vi "MODBUS  SLAVE.vi"() -> (3 "values to write":u16[](array[numeric]) caption="待写入值")   [LabVIEW 2016]
uses:
  <vilib>/NI/Modbus Library/Data Model/Device Data Model.lvclass
  <vilib>/NI/Modbus Library/API/Wrapper/Create TCP Slave.vi
  <vilib>/NI/Modbus Library/API/Slave/Modbus Slave.lvclass
  <vilib>/ptbypt/NI_PtbyPt.lvlib
  <vilib>/NI/Modbus Library/API/Wrapper/API Main.lvlib
panel:
  out "运行周期":u16[](array[numeric])
  in  "write operation starting address":u16=100 caption="写操作起始地址"
  out "单仪器启动命令":u16[](array[numeric])
  out "系统启动命令":u16[](array[numeric])
  in  "停止":bool
  out "register values":u16[](array[numeric]) caption="寄存器值"
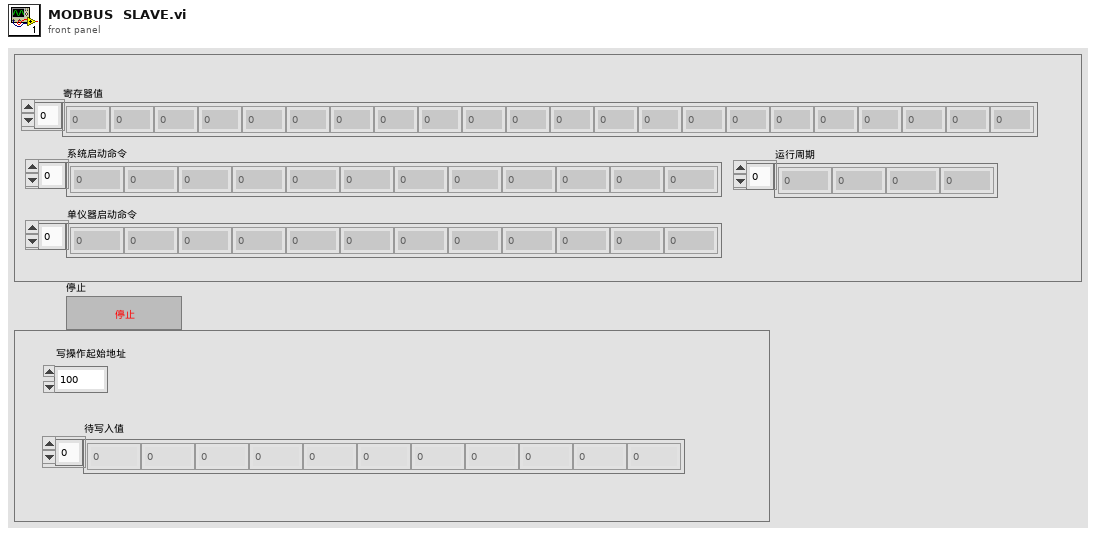
[diagram p1: front panel]
types:
  T1 = cluster{"测量模式":enum16{"水样测量", "标样核查", "零点核查", "跨度核查", "空白测试", "加标回收", "平行样", "校零", "校标"}}
  T2 = cluster{"站号":u16, "量程切换":enum32{"H", "L", "AUTO"}, "控制命令":enum16{"启动测量", "标样核查", "零点核查", "跨度核查", "空白测试", "平行样测试", "加标回收", "空白校准", "标样校准", "初始化（清洗）", "停止测试", "仪器重启", "校时", "模式设置", "测量间隔设置"}, "模式设置":enum16{"待机", "连续模式", "周期模式", "定点模式", "受控模式", "手动模式"}, "测量间隔":u16}
  T3 = cluster{"系统时间":timestamp, "工作状态":enum16{"空闲", "水样测试", "标样核查", "零点核查", "跨度核查", "空白测试", "平行样测试", "加标回收", "空白校准", "标样校准", "初始化（清洗）"}, "测量模式":enum16{"待机", "连续模式", "周期模式", "定点模式", "受控模式", "手动模式"}, "告警代码":enum16{"无告警", "缺试剂告警", "缺水样告警", "缺蒸馏水告警", "缺标液告警", "仪表漏液告警", "标定异常告警", "超量程告警", "加热异常", "低试剂预警", "超上限告警", "超下限告警", "仪表内部其他异常", "滴定异常告警", "电极异常告警", "量程切换告警", "参数设置告警", "PH电极电位异常", "电导率电极异常", "浊度光度异常", "溶解氧电极异常", "溶解氧光强异常", "温度异常告警", "PH异常告警", "溶解氧异常告警", "电导率异常告警", "浊度异常告警", "叶绿素异常告警", "藻密度异常告警", "蓝绿藻异常告警", "ORP异常告警", "氨氮异常告警", "清洁刷异常告警", "SD卡异常告警", "蓝牙异常告警", "Wifi异常告警", "流程异常告警"}, "故障代码":enum16{"无故障", "电机故障", "温度故障", "通讯故障", "滴定故障"}, "日志代码":u16, "软件版本":u16, "F0":sgl, "F1":sgl, "F2":sgl, "F3":sgl, "T":sgl, "H":sgl, "id":u16, "flowid":u16, "量程":u16, "总磷控温温度1":sgl, "营养盐控温温度2":sgl, "ADC":sgl}
  T4 = enum16{"空闲", "水样测试", "标样核查", "零点核查", "跨度核查", "空白测试", "平行样测试", "质控样", "空白校准", "标样校准", "加标回收"}
  T5 = cluster{"当前瓶号：":dbl, "平行样：":dbl, "留样瓶数：":dbl, "每瓶次数：":dbl, "每次留样：":dbl}
  T6 = enum16{"空闲", "水样测试", "标样核查", "零点核查", "跨度核查", "空白测试", "平行样测试", "加标回收", "空白校准", "标样校准", "初始化（清洗）"}
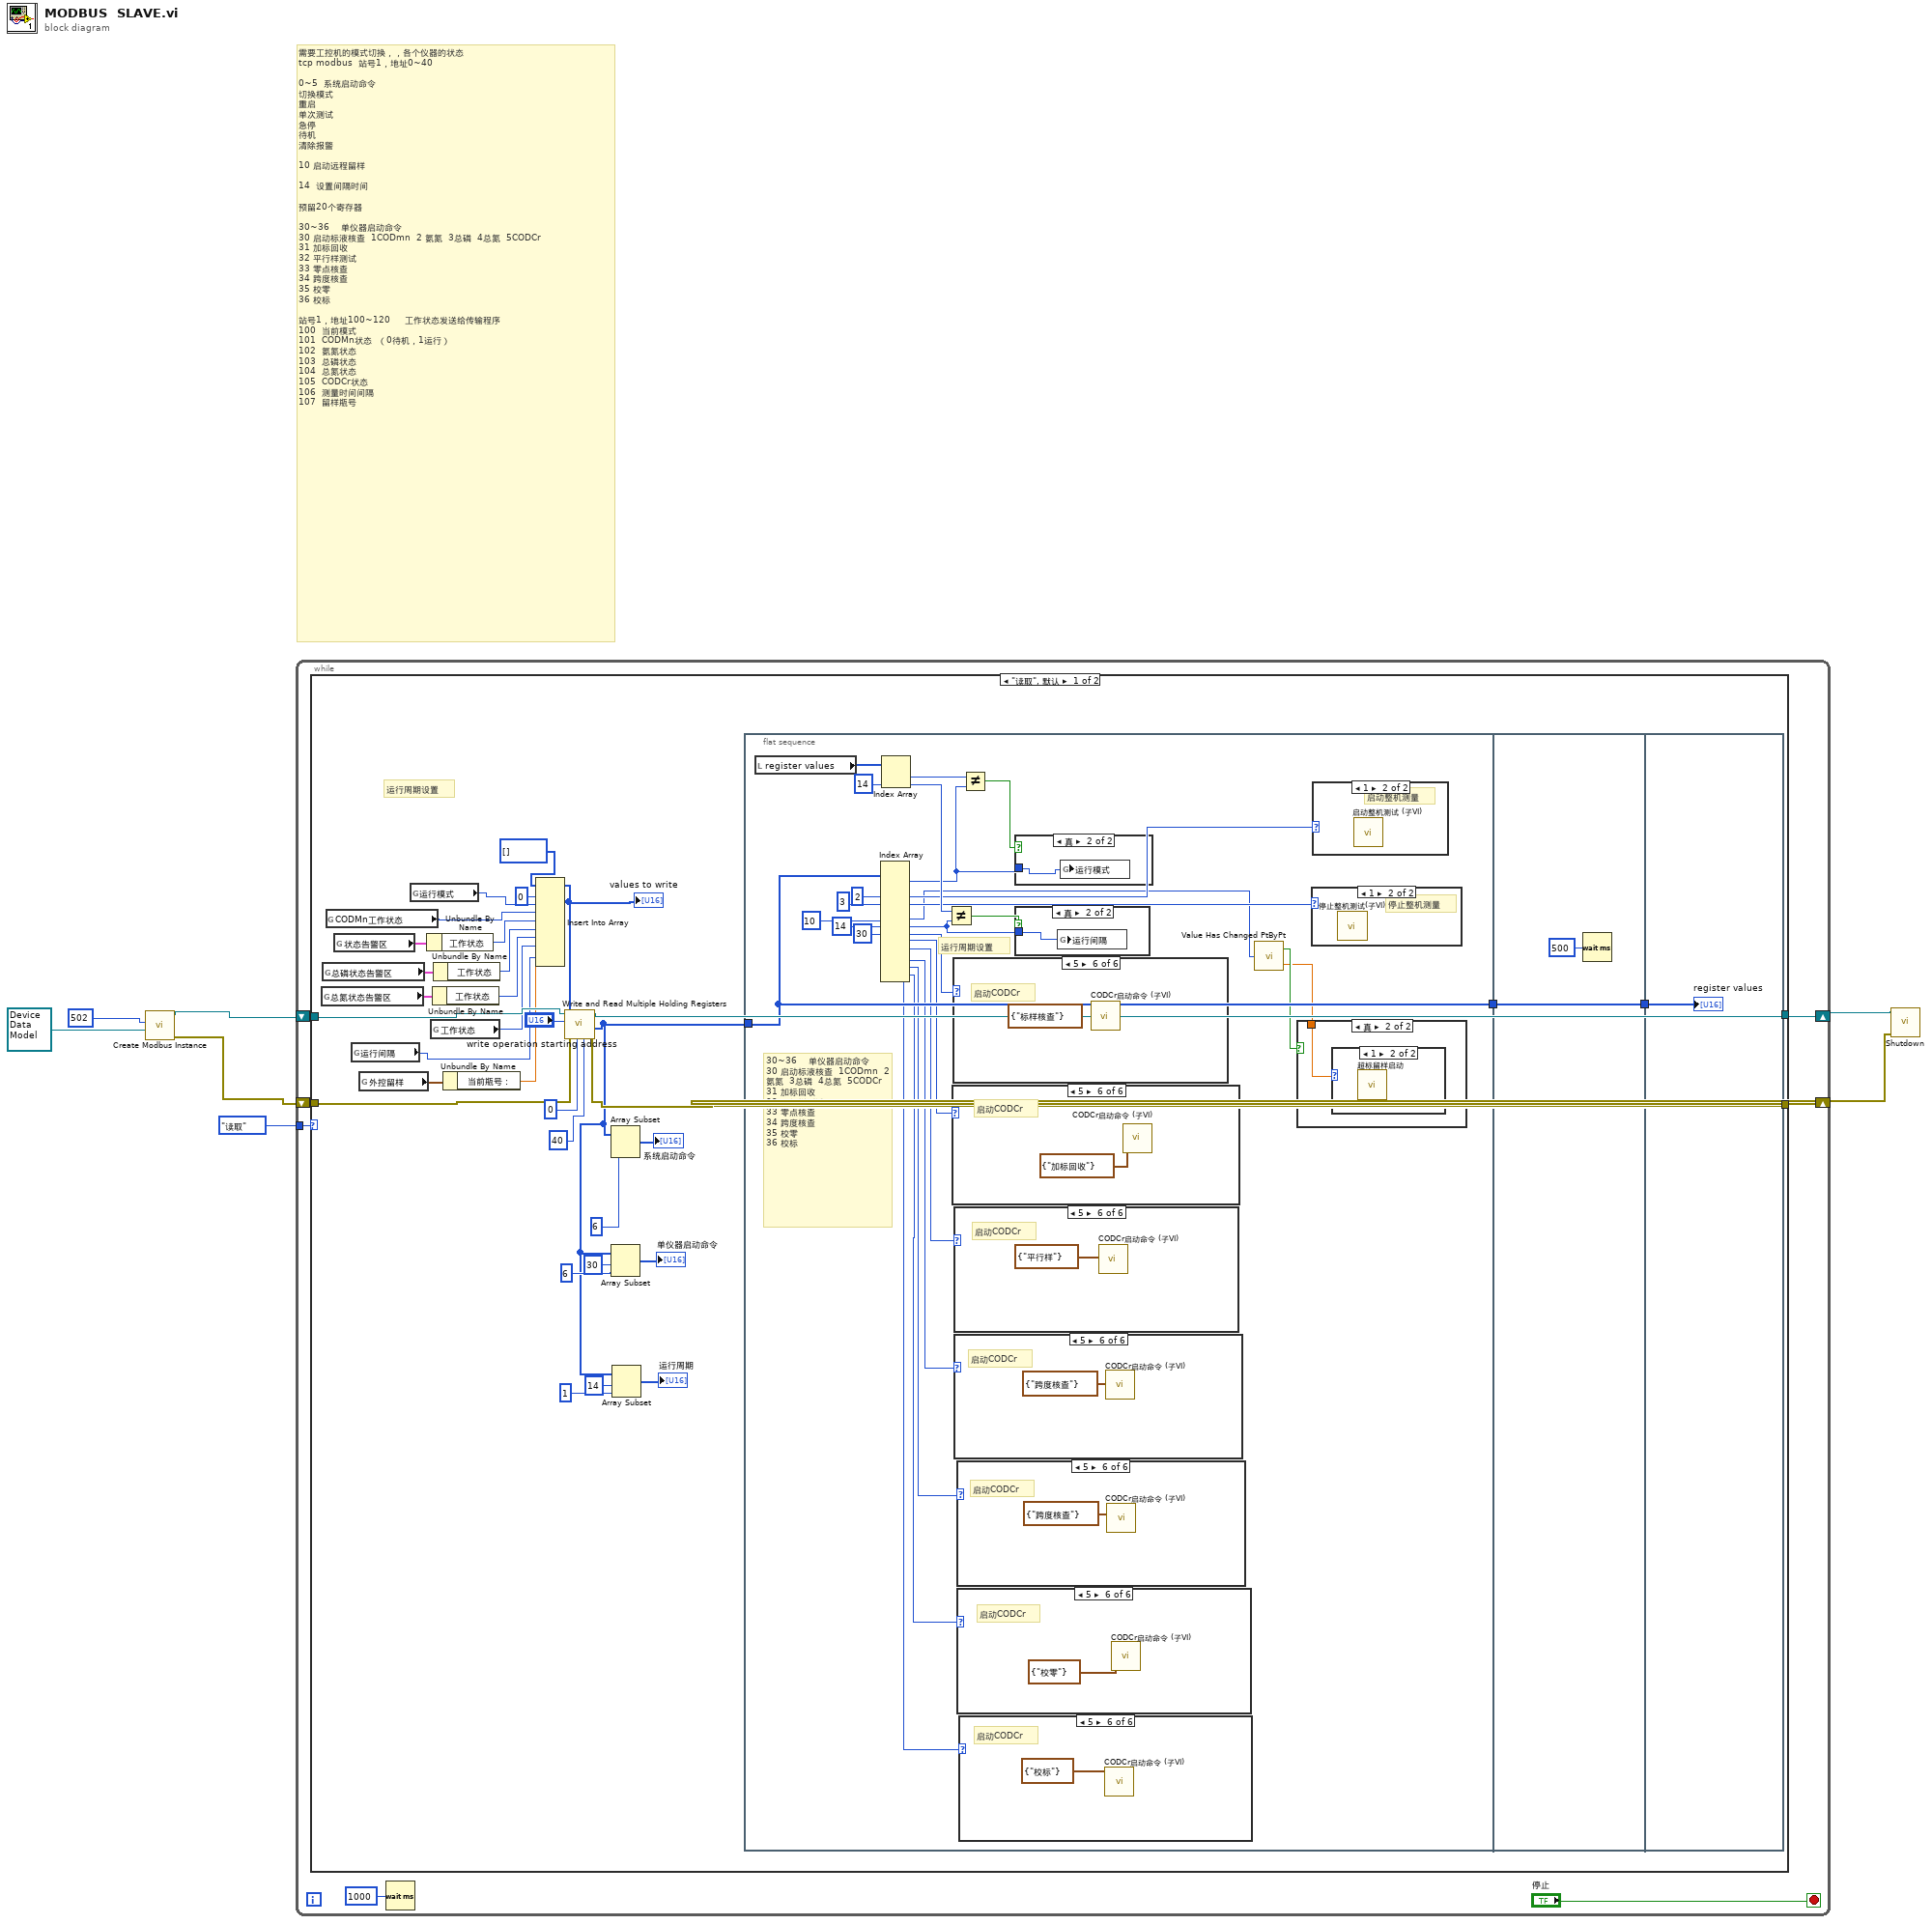
[diagram p0: block diagram]
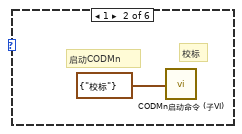
[diagram p5: hidden frame]
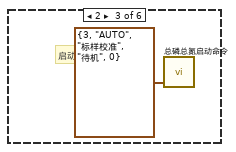
[diagram p6: hidden frame]
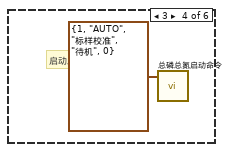
[diagram p7: hidden frame]
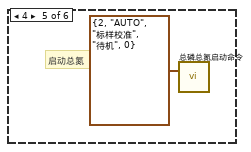
[diagram p8: hidden frame]
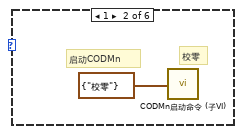
[diagram p10: hidden frame]
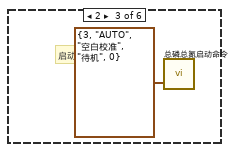
[diagram p11: hidden frame]
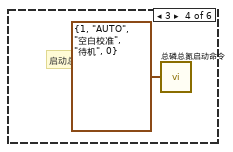
[diagram p12: hidden frame]
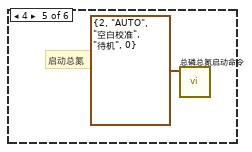
[diagram p13: hidden frame]
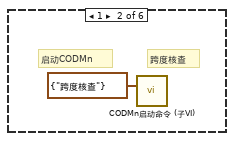
[diagram p15: hidden frame]
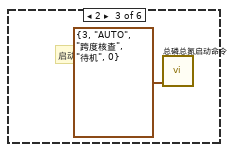
[diagram p16: hidden frame]
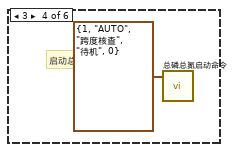
[diagram p17: hidden frame]
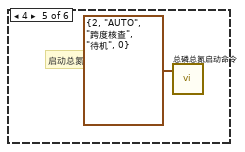
[diagram p18: hidden frame]
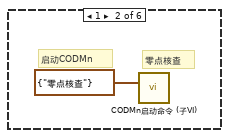
[diagram p20: hidden frame]
diagram:
  # "需要工控机的模式切换，，各个仪器的状态\ntcp modbus  站号1，地址0~40\n\n0~5  系统启动命令\n切换模式\n重启\n单次测试\n急停\n待机\n清除报警\n\n10 启动远程留样\n\n14  设置间隔时间\n\n预留20个寄存器\n\n30~36    单仪器启动命令\n30 启动标液核查  1CODmn  2 氨氮  3总磷  4总氮  5CODCr\n31 加标回收\n32 平行样测试\n33 零点核查\n34 跨度核查\n35 校零\n36 校标\n\n站号1，地址100~120     工作状态发送给传输程序\n100  当前模式\n101  CODMn状态  （0待机，1运行）\n102  氨氮状态\n103  总磷状态\n104  总氮状态\n105  CODCr状态\n106  测量时间间隔\n107  留样瓶号"
  n1 = call-poly <vilib>:"Create Modbus Instance.vi"("device data model"=refnum<class "Device Data Model.lvclass"> refnum, "port (502)"=u16 502) -> ("error out"=w5:errorcluster, "TCP slave instance"=w6:refnum<class "Modbus Slave.lvclass">)  [unwired: 8 in]
  n2 = while {
    shift-right: [w12] -> w2
    shift-left: w6 -> [w14]
    shift-right: [w8] -> w1
    shift-left: w5 -> [w13]
    tunnel: enum16{"读取", "写入"}."读取" -> [w9]
    stop <- "停止" stop-if-true
    n3 = case shown="\"读取\", 默认" w9 {
      tunnel: w14 -> [w43 w116]
      tunnel: w13 -> [w42 w115]
      tunnel: [w38 w116] -> w12
      tunnel: [w39 w115] -> w8
      frame "读取", Default {
        # "运行周期设置"
        n4 = global read "VAR总磷总氮全局变量.vi" "总氮状态告警区"() -> (w22:T3)
        n5 = global read "VAR总磷总氮全局变量.vi" "总磷状态告警区"() -> (w24:T3)
        n6 = global read "COD测量模式全局.vi" "CODMn工作状态"() -> (w20:T4)
        n7 = global read "VAR氨氮全局变量.vi" "状态告警区"() -> (w26:T3)
        n8 = global read "系统设置全局变量.vi" "运行间隔"() -> (w16:i16)
        n9 = global read "超标留样全局.vi" "外控留样"() -> (w18:T5)
        n10 = global read "系统设置全局变量.vi" "运行模式"() -> (w15:enum16{"维护模式", "常规模式", "应急模式", "质控模式"})
        n11 = Unbundle By Name(w26) -> ("工作状态"=w25:T6)
        n12 = global read "CODcr全局变量.vi" "工作状态"() -> (w19:T6)
        n13 = Unbundle By Name(w22) -> ("工作状态"=w21:T6)
        n14 = Unbundle By Name(w24) -> ("工作状态"=w23:T6)
        n15 = Unbundle By Name(w18) -> ("当前瓶号："=w17:dbl)
        n16 = Insert Into Array(array=u16[] [] ("values to write"), index=0 ("索引"), new element #1=w15, new element #2=w20, new element #3=w25, new element #4=w23, new element #5=w21, new element #6=w19, new element #7=w16, new element #8=w17) -> (w34:u16[])
        "values to write" <- w34
        n17 = call-dynamic "Write and Read Multiple Holding Registers.vi"("read count"=u16 40 ("number of holding registers"), "read starting address"=u16 0 ("starting address"), "error in"=w42, "write values"=w34, "write starting address"="write operation starting address", "Modbus instance in"=w43) -> ("error out"=w39:errorcluster, "read values"=w29:u16[], "Modbus instance out"=w38:refnum<class "Modbus Slave.lvclass">)  [unwired: 3 in]
        n18 = Array Subset(array=w29, length=6 ("长度")) -> (→"系统启动命令":u16[])  [unwired: 1 in]
        n19 = Array Subset(array=w29, index=30 ("索引"), length=6 ("长度")) -> (→"单仪器启动命令":u16[])
        n20 = Array Subset(array=w29, index=14 ("索引"), length=1 ("长度")) -> (→"运行周期":u16[])
        n21 = flat-sequence {
          tunnel: w29 -> [w73]
          tunnel: [w73] -> w28
          tunnel: w28 -> [w112]
          tunnel: [w112] -> w27
          tunnel: w27 -> [w114]
          frame #0 {
            # "运行周期设置"
            # "30~36    单仪器启动命令\n30 启动标液核查  1CODmn  2 氨氮  3总磷  4总氮  5CODCr\n31 加标回收\n32 平行样测试\n33 零点核查\n34 跨度核查\n35 校零\n36 校标"
            n22 = local read "register values"() -> (w72:u16[])
            n23 = Index Array(array=w73, index #3=2 ("索引"), index #4=3 ("索引"), index #6=10 ("索引"), index #7=14 ("索引"), index #8=30 ("索引")) -> (element #1=w60:u16, element #3=w61:u16, element #4=w62:u16, element #6=w50:u16, element #7=w63:u16, element #8=w58:u16, element #9=w57:u16, element #10=w56:u16, element #11=w55:u16, element #12=w54:u16, element #13=w53:u16, element #14=w52:u16)  [unwired: 9 in, 2 out]
            n24 = Index Array(array=w72, index #2=14 ("索引")) -> (element #1=w71:u16, element #2=w68:u16)  [unwired: 1 in]
            n25 = Not Equal?(x=w68, y=w63) -> (x != y?=w67:bool)
            n26 = case shown="5" w57 {
              frame 0, Default {
              }
              frame 1 {
                # "加标回收"
                # "启动CODMn"
                n27 = call "CODMn启动命令 (子VI).vi"("启动测量模式"=T1 {"测量模式"=enum."加标回收"}) -> ()  [unwired: 11 in]
              }
              frame 2 {
                # "启动氨氮"
                n28 = call "总磷总氮启动命令.vi"("参数"=T2 {"站号"=3, "量程切换"=enum."AUTO", "控制命令"=enum."加标回收", "模式设置"=enum."待机", "测量间隔"=0}) -> ()  [unwired: 10 in, 1 out]
              }
              frame 3 {
                # "启动总磷"
                n29 = call "总磷总氮启动命令.vi"("参数"=T2 {"站号"=1, "量程切换"=enum."AUTO", "控制命令"=enum."加标回收", "模式设置"=enum."待机", "测量间隔"=0}) -> ()  [unwired: 10 in, 1 out]
              }
              frame 4 {
                # "启动总氮"
                n30 = call "总磷总氮启动命令.vi"("参数"=T2 {"站号"=2, "量程切换"=enum."AUTO", "控制命令"=enum."加标回收", "模式设置"=enum."待机", "测量间隔"=0}) -> ()  [unwired: 10 in, 1 out]
              }
              frame 5 {
                # "启动CODCr"
                n31 = call "CODCr启动命令 (子VI).vi"("启动测量模式"=T1 {"测量模式"=enum."加标回收"}) -> ()  [unwired: 11 in]
              }
            }
            n32 = case shown="5" w58 {
              frame 0, Default {
              }
              frame 1 {
                # "启动标液核查"
                # "启动CODMn"
                n33 = call "CODMn启动命令 (子VI).vi"("启动测量模式"=T1 {"测量模式"=enum."标样核查"}) -> ()  [unwired: 11 in]
              }
              frame 2 {
                # "启动氨氮"
                n34 = call "总磷总氮启动命令.vi"("参数"=T2 {"站号"=3, "量程切换"=enum."AUTO", "控制命令"=enum."标样核查", "模式设置"=enum."待机", "测量间隔"=0}) -> ()  [unwired: 10 in, 1 out]
              }
              frame 3 {
                # "启动总磷"
                n35 = call "总磷总氮启动命令.vi"("参数"=T2 {"站号"=1, "量程切换"=enum."AUTO", "控制命令"=enum."标样核查", "模式设置"=enum."待机", "测量间隔"=0}) -> ()  [unwired: 10 in, 1 out]
              }
              frame 4 {
                # "启动总氮"
                n36 = call "总磷总氮启动命令.vi"("参数"=T2 {"站号"=2, "量程切换"=enum."AUTO", "控制命令"=enum."标样核查", "模式设置"=enum."待机", "测量间隔"=0}) -> ()  [unwired: 10 in, 1 out]
              }
              frame 5 {
                # "启动CODCr"
                n37 = call "CODCr启动命令 (子VI).vi"("启动测量模式"=T1 {"测量模式"=enum."标样核查"}) -> ()  [unwired: 11 in]
              }
            }
            n38 = case shown="5" w56 {
              frame 0, Default {
              }
              frame 1 {
                # "平行样测试"
                # "启动CODMn"
                n39 = call "CODMn启动命令 (子VI).vi"("启动测量模式"=T1 {"测量模式"=enum."平行样"}) -> ()  [unwired: 11 in]
              }
              frame 2 {
                # "启动氨氮"
                n40 = call "总磷总氮启动命令.vi"("参数"=T2 {"站号"=3, "量程切换"=enum."AUTO", "控制命令"=enum."平行样测试", "模式设置"=enum."待机", "测量间隔"=0}) -> ()  [unwired: 10 in, 1 out]
              }
              frame 3 {
                # "启动总磷"
                n41 = call "总磷总氮启动命令.vi"("参数"=T2 {"站号"=1, "量程切换"=enum."AUTO", "控制命令"=enum."平行样测试", "模式设置"=enum."待机", "测量间隔"=0}) -> ()  [unwired: 10 in, 1 out]
              }
              frame 4 {
                # "启动总氮"
                n42 = call "总磷总氮启动命令.vi"("参数"=T2 {"站号"=2, "量程切换"=enum."AUTO", "控制命令"=enum."平行样测试", "模式设置"=enum."待机", "测量间隔"=0}) -> ()  [unwired: 10 in, 1 out]
              }
              frame 5 {
                # "启动CODCr"
                n43 = call "CODCr启动命令 (子VI).vi"("启动测量模式"=T1 {"测量模式"=enum."平行样"}) -> ()  [unwired: 11 in]
              }
            }
            n44 = case shown="5" w55 {
              frame 0, Default {
              }
              frame 1 {
                # "零点核查"
                # "启动CODMn"
                n45 = call "CODMn启动命令 (子VI).vi"("启动测量模式"=T1 {"测量模式"=enum."零点核查"}) -> ()  [unwired: 11 in]
              }
              frame 2 {
                # "启动氨氮"
                n46 = call "总磷总氮启动命令.vi"("参数"=T2 {"站号"=3, "量程切换"=enum."AUTO", "控制命令"=enum."零点核查", "模式设置"=enum."待机", "测量间隔"=0}) -> ()  [unwired: 10 in, 1 out]
              }
              frame 3 {
                # "启动总磷"
                n47 = call "总磷总氮启动命令.vi"("参数"=T2 {"站号"=1, "量程切换"=enum."AUTO", "控制命令"=enum."零点核查", "模式设置"=enum."待机", "测量间隔"=0}) -> ()  [unwired: 10 in, 1 out]
              }
              frame 4 {
                # "启动总氮"
                n48 = call "总磷总氮启动命令.vi"("参数"=T2 {"站号"=2, "量程切换"=enum."AUTO", "控制命令"=enum."零点核查", "模式设置"=enum."待机", "测量间隔"=0}) -> ()  [unwired: 10 in, 1 out]
              }
              frame 5 {
                # "启动CODCr"
                n49 = call "CODCr启动命令 (子VI).vi"("启动测量模式"=T1 {"测量模式"=enum."跨度核查"}) -> ()  [unwired: 11 in]
              }
            }
            n50 = case shown="5" w54 {
              frame 0, Default {
              }
              frame 1 {
                # "跨度核查"
                # "启动CODMn"
                n51 = call "CODMn启动命令 (子VI).vi"("启动测量模式"=T1 {"测量模式"=enum."跨度核查"}) -> ()  [unwired: 11 in]
              }
              frame 2 {
                # "启动氨氮"
                n52 = call "总磷总氮启动命令.vi"("参数"=T2 {"站号"=3, "量程切换"=enum."AUTO", "控制命令"=enum."跨度核查", "模式设置"=enum."待机", "测量间隔"=0}) -> ()  [unwired: 10 in, 1 out]
              }
              frame 3 {
                # "启动总磷"
                n53 = call "总磷总氮启动命令.vi"("参数"=T2 {"站号"=1, "量程切换"=enum."AUTO", "控制命令"=enum."跨度核查", "模式设置"=enum."待机", "测量间隔"=0}) -> ()  [unwired: 10 in, 1 out]
              }
              frame 4 {
                # "启动总氮"
                n54 = call "总磷总氮启动命令.vi"("参数"=T2 {"站号"=2, "量程切换"=enum."AUTO", "控制命令"=enum."跨度核查", "模式设置"=enum."待机", "测量间隔"=0}) -> ()  [unwired: 10 in, 1 out]
              }
              frame 5 {
                # "启动CODCr"
                n55 = call "CODCr启动命令 (子VI).vi"("启动测量模式"=T1 {"测量模式"=enum."跨度核查"}) -> ()  [unwired: 11 in]
              }
            }
            n56 = case shown="5" w53 {
              frame 0, Default {
              }
              frame 1 {
                # "校零"
                # "启动CODMn"
                n57 = call "CODMn启动命令 (子VI).vi"("启动测量模式"=T1 {"测量模式"=enum."校零"}) -> ()  [unwired: 11 in]
              }
              frame 2 {
                # "启动氨氮"
                n58 = call "总磷总氮启动命令.vi"("参数"=T2 {"站号"=3, "量程切换"=enum."AUTO", "控制命令"=enum."空白校准", "模式设置"=enum."待机", "测量间隔"=0}) -> ()  [unwired: 10 in, 1 out]
              }
              frame 3 {
                # "启动总磷"
                n59 = call "总磷总氮启动命令.vi"("参数"=T2 {"站号"=1, "量程切换"=enum."AUTO", "控制命令"=enum."空白校准", "模式设置"=enum."待机", "测量间隔"=0}) -> ()  [unwired: 10 in, 1 out]
              }
              frame 4 {
                # "启动总氮"
                n60 = call "总磷总氮启动命令.vi"("参数"=T2 {"站号"=2, "量程切换"=enum."AUTO", "控制命令"=enum."空白校准", "模式设置"=enum."待机", "测量间隔"=0}) -> ()  [unwired: 10 in, 1 out]
              }
              frame 5 {
                # "启动CODCr"
                n61 = call "CODCr启动命令 (子VI).vi"("启动测量模式"=T1 {"测量模式"=enum."校零"}) -> ()  [unwired: 11 in]
              }
            }
            n62 = case shown="5" w52 {
              frame 0, Default {
              }
              frame 1 {
                # "校标"
                # "启动CODMn"
                n63 = call "CODMn启动命令 (子VI).vi"("启动测量模式"=T1 {"测量模式"=enum."校标"}) -> ()  [unwired: 11 in]
              }
              frame 2 {
                # "启动氨氮"
                n64 = call "总磷总氮启动命令.vi"("参数"=T2 {"站号"=3, "量程切换"=enum."AUTO", "控制命令"=enum."标样校准", "模式设置"=enum."待机", "测量间隔"=0}) -> ()  [unwired: 10 in, 1 out]
              }
              frame 3 {
                # "启动总磷"
                n65 = call "总磷总氮启动命令.vi"("参数"=T2 {"站号"=1, "量程切换"=enum."AUTO", "控制命令"=enum."标样校准", "模式设置"=enum."待机", "测量间隔"=0}) -> ()  [unwired: 10 in, 1 out]
              }
              frame 4 {
                # "启动总氮"
                n66 = call "总磷总氮启动命令.vi"("参数"=T2 {"站号"=2, "量程切换"=enum."AUTO", "控制命令"=enum."标样校准", "模式设置"=enum."待机", "测量间隔"=0}) -> ()  [unwired: 10 in, 1 out]
              }
              frame 5 {
                # "启动CODCr"
                n67 = call "CODCr启动命令 (子VI).vi"("启动测量模式"=T1 {"测量模式"=enum."校标"}) -> ()  [unwired: 11 in]
              }
            }
            n68 = Not Equal?(x=w71, y=w60) -> (x != y?=w70:bool)
            n69 = case shown="真" w70 {
              tunnel: w60 -> [_ w111]
              frame False {
              }
              frame True {
                n70 = global write "系统设置全局变量.vi" "运行模式"(w111) -> ()
              }
            }
            n71 = case shown="真" w67 {
              tunnel: w63 -> [_ w110]
              frame False {
              }
              frame True {
                n72 = global write "系统设置全局变量.vi" "运行间隔"(w110) -> ()
              }
            }
            n73 = call <vilib>:"Value Has Changed PtByPt.vi"("input data point"=w50) -> ("has changed"=w49:bool, "output data point"=w48:dbl)  [unwired: 1 in]
            n74 = case shown="真" w49 {
              tunnel: w48 -> [_ w74]
              frame False {
              }
              frame True {
                n75 = case shown="1" w74 {
                  frame 0, Default {
                  }
                  frame 1 {
                    n76 = call "超标留样启动.vi"() -> ()  [unwired: 11 in, 1 out]
                  }
                }
              }
            }
            n77 = case shown="1" w62 {
              frame 0, Default {
              }
              frame 1 {
                # "停止整机测量"
                n78 = call "停止整机测试(子VI).vi"() -> ()  [unwired: 12 in]
              }
            }
            n79 = case shown="1" w61 {
              frame 0, Default {
              }
              frame 1 {
                # "启动整机测量"
                n80 = call "启动整机测试 (子VI).vi"() -> ()  [unwired: 12 in]
              }
            }
          }
          frame #1 {
            n81 = Wait (ms)(milliseconds to wait=u32 500 ("等待时间（毫秒）")) -> ()  [unwired: 1 out]
          }
          frame #2 {
            "register values" <- w114
          }
        }
      }
      frame "写入" {
      }
    }
    n82 = Wait (ms)(milliseconds to wait=u32 1000 ("等待时间（毫秒）")) -> ()  [unwired: 1 out]
  }
  n83 = call-dynamic "Shutdown.vi"("error in"=w1, "Modbus slave in"=w2) -> ()  [unwired: 9 in, 1 out]
